vi "FA Values View2.vi"(11 "Model in":refnum<class "Model.lvclass">) -> ()   [LabVIEW 2016, in "M1M3SupportEUI_Views.lvlib"]
uses:
  M1M3SupportEUI_Views.lvlib
  Model/Model.lvclass
  SALLV_m1m3/DataTypes/ForceActuatorData.ctl
  SALLV_m1m3/DataTypes/logevent_ForceActuatorInfo.ctl
  SALLV_m1m3/DataTypes/logevent_ForceActuatorState.ctl
  SALLV_m1m3/DataTypes/logevent_ForceActuatorWarning.ctl
  SALLV_m1m3/DataTypes/logevent_ForceSetpointWarning.ctl
  SALLV_m1m3/DataTypes/logevent_ForceActuatorForceWarning.ctl
  SALLV_m1m3/DataTypes/logevent_AppliedAberrationForces.ctl
  SALLV_m1m3/DataTypes/logevent_AppliedAccelerationForces.ctl
  SALLV_m1m3/DataTypes/logevent_AppliedActiveOpticForces.ctl
  SALLV_m1m3/DataTypes/logevent_AppliedAzimuthForces.ctl
  SALLV_m1m3/DataTypes/logevent_AppliedBalanceForces.ctl
  SALLV_m1m3/DataTypes/logevent_AppliedCylinderForces.ctl
  SALLV_m1m3/DataTypes/logevent_AppliedElevationForces.ctl
  SALLV_m1m3/DataTypes/logevent_AppliedForces.ctl
  SALLV_m1m3/DataTypes/logevent_AppliedOffsetForces.ctl
  SALLV_m1m3/DataTypes/logevent_AppliedStaticForces.ctl
  SALLV_m1m3/DataTypes/logevent_AppliedThermalForces.ctl
  SALLV_m1m3/DataTypes/logevent_AppliedVelocityForces.ctl
  SALLV_m1m3/DataTypes/logevent_RejectedAberrationForces.ctl
  SALLV_m1m3/DataTypes/logevent_RejectedAccelerationForces.ctl
  SALLV_m1m3/DataTypes/logevent_RejectedActiveOpticForces.ctl
  SALLV_m1m3/DataTypes/logevent_RejectedAzimuthForces.ctl
  SALLV_m1m3/DataTypes/logevent_RejectedBalanceForces.ctl
  SALLV_m1m3/DataTypes/logevent_RejectedCylinderForces.ctl
  SALLV_m1m3/DataTypes/logevent_RejectedElevationForces.ctl
  SALLV_m1m3/DataTypes/logevent_RejectedForces.ctl
  SALLV_m1m3/DataTypes/logevent_RejectedOffsetForces.ctl
  SALLV_m1m3/DataTypes/logevent_RejectedStaticForces.ctl
  SALLV_m1m3/DataTypes/logevent_RejectedThermalForces.ctl
  SALLV_m1m3/DataTypes/logevent_RejectedVelocityForces.ctl
  M1M3 Support Events/M1M3 Support Events.lvclass/M1M3 Support Events.ctl
  M1M3 Support Events/M1M3 Support Events.lvclass
  SALLV_m1m3/SALLV_m1m3.lvlib
panel:
  out "Numeric":i32
  out "Timestamp":timestamp
  in  "logevent_RejectedVelocityForces":T1
  in  "logevent_RejectedThermalForces":T2
  in  "logevent_RejectedStaticForces":T3
  in  "logevent_RejectedOffsetForces":T4
  in  "logevent_RejectedForces":T5
  in  "logevent_RejectedElevationForces":T6
  in  "logevent_RejectedCylinderForces":T7
  in  "logevent_RejectedBalanceForces":T8
  in  "logevent_RejectedAzimuthForces":T9
  in  "logevent_RejectedActiveOpticForces":T10
  in  "logevent_RejectedAccelerationForces":T11
  in  "logevent_RejectedAberrationForces":T12
  in  "logevent_AppliedVelocityForces":T13
  in  "logevent_AppliedThermalForces":T14
  in  "logevent_AppliedStaticForces":T15
  in  "logevent_AppliedOffsetForces":T16
  in  "logevent_AppliedForces":T17
  in  "logevent_AppliedElevationForces":T18
  in  "logevent_AppliedCylinderForces":T19
  in  "logevent_AppliedBalanceForces":T20
  in  "logevent_AppliedAzimuthForces":T21
  in  "logevent_AppliedActiveOpticForces":T22
  in  "logevent_AppliedAccelerationForces":T23
  in  "logevent_AppliedAberrationForces":T24
  in  "logevent_ForceActuatorForceWarning":T25
  in  "logevent_ForceSetpointWarning":T26
  in  "logevent_ForceActuatorWarning":T27
  in  "logevent_ForceActuatorState":T28
  out "logevent_ForceActuatorInfo":T29
  out "ForceActuatorData":T30 {"Timestamp" format="%#_14f"}
  in  "Field":string(combo)
  out "Display":string[][](array[string])
  out "stop":bool
  in  "Topic":string(combo)
  # "Force Actuators"
  # "0"
  # "1"
  # "2"
  # "3"
  # "4"
  # "5"
  # "6"
  # "7"
  # "8"
  # "9"
  # "100"
  # "110"
  # "120"
  # "130"
  # "140"
  # "200"
  # "210"
  # "220"
  # "230"
  # "240"
  # "300"
  # "310"
  # "320"
  # "330"
  # "340"
  # "400"
  # "410"
  # "420"
  # "430"
  # "440"
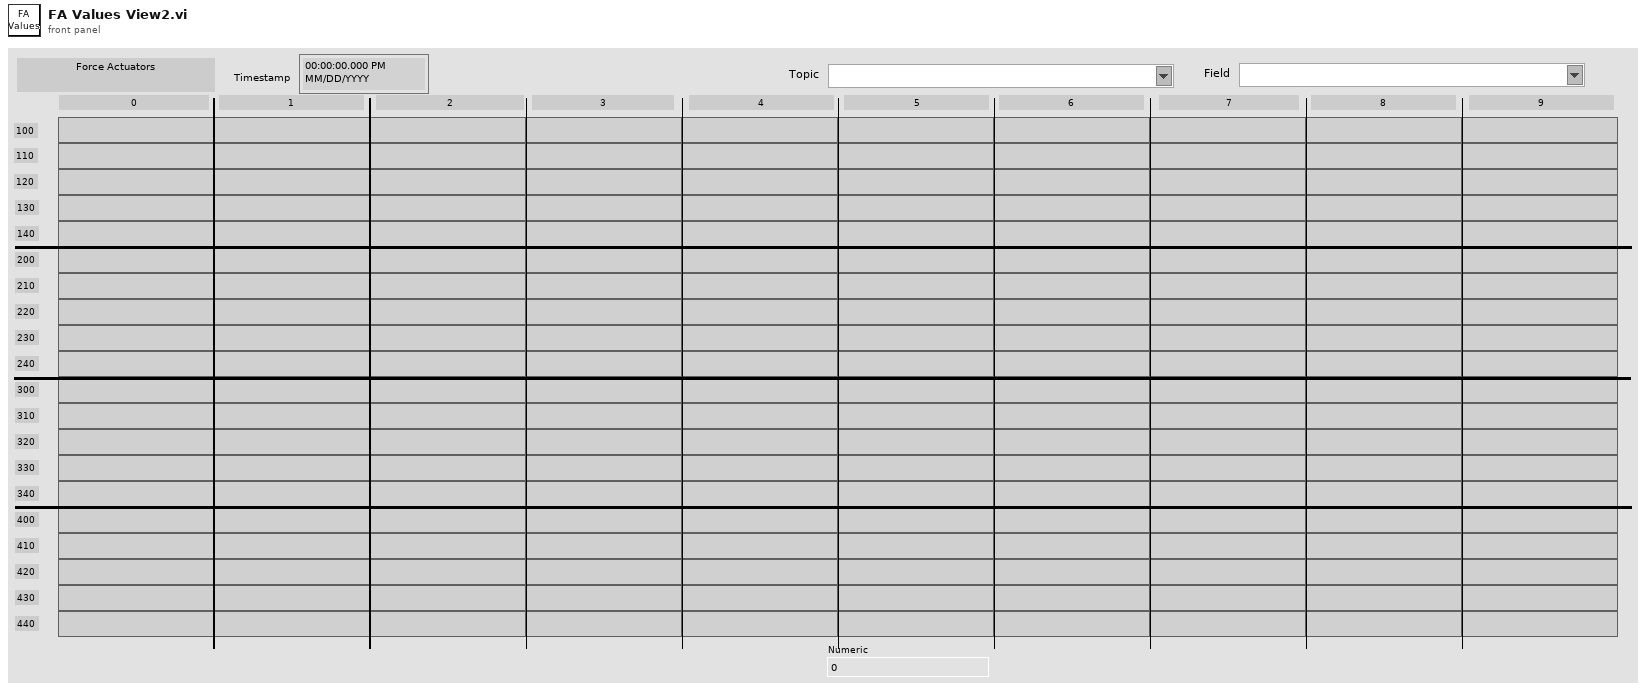
[diagram p1: front panel]
types:
  T1 = typedef "SALLV_m1m3.lvlib/logevent_RejectedVelocityForces.ctl" = cluster{"Timestamp":dbl, "XForces[12]":sgl[], "YForces[100]":sgl[], "ZForces[156]":sgl[], "Fx":sgl, "Fy":sgl, "Fz":sgl, "Mx":sgl, "My":sgl, "Mz":sgl, "ForceMagnitude":sgl, "priority":i32}
  T2 = typedef "SALLV_m1m3.lvlib/logevent_RejectedThermalForces.ctl" = cluster{"Timestamp":dbl, "XForces[12]":sgl[], "YForces[100]":sgl[], "ZForces[156]":sgl[], "Fx":sgl, "Fy":sgl, "Fz":sgl, "Mx":sgl, "My":sgl, "Mz":sgl, "ForceMagnitude":sgl, "priority":i32}
  T3 = typedef "SALLV_m1m3.lvlib/logevent_RejectedStaticForces.ctl" = cluster{"Timestamp":dbl, "XForces[12]":sgl[], "YForces[100]":sgl[], "ZForces[156]":sgl[], "Fx":sgl, "Fy":sgl, "Fz":sgl, "Mx":sgl, "My":sgl, "Mz":sgl, "ForceMagnitude":sgl, "priority":i32}
  T4 = typedef "SALLV_m1m3.lvlib/logevent_RejectedOffsetForces.ctl" = cluster{"Timestamp":dbl, "XForces[12]":sgl[], "YForces[100]":sgl[], "ZForces[156]":sgl[], "Fx":sgl, "Fy":sgl, "Fz":sgl, "Mx":sgl, "My":sgl, "Mz":sgl, "ForceMagnitude":sgl, "priority":i32}
  T5 = typedef "SALLV_m1m3.lvlib/logevent_RejectedForces.ctl" = cluster{"Timestamp":dbl, "XForces[12]":sgl[], "YForces[100]":sgl[], "ZForces[156]":sgl[], "Fx":sgl, "Fy":sgl, "Fz":sgl, "Mx":sgl, "My":sgl, "Mz":sgl, "ForceMagnitude":sgl, "priority":i32}
  T6 = typedef "SALLV_m1m3.lvlib/logevent_RejectedElevationForces.ctl" = cluster{"Timestamp":dbl, "XForces[12]":sgl[], "YForces[100]":sgl[], "ZForces[156]":sgl[], "Fx":sgl, "Fy":sgl, "Fz":sgl, "Mx":sgl, "My":sgl, "Mz":sgl, "ForceMagnitude":sgl, "priority":i32}
  T7 = typedef "SALLV_m1m3.lvlib/logevent_RejectedCylinderForces.ctl" = cluster{"Timestamp":dbl, "SecondaryCylinderForces[112]":i32[], "PrimaryCylinderForces[156]":i32[], "priority":i32}
  T8 = typedef "SALLV_m1m3.lvlib/logevent_RejectedBalanceForces.ctl" = cluster{"Timestamp":dbl, "XForces[12]":sgl[], "YForces[100]":sgl[], "ZForces[156]":sgl[], "Fx":sgl, "Fy":sgl, "Fz":sgl, "Mx":sgl, "My":sgl, "Mz":sgl, "ForceMagnitude":sgl, "priority":i32}
  T9 = typedef "SALLV_m1m3.lvlib/logevent_RejectedAzimuthForces.ctl" = cluster{"Timestamp":dbl, "XForces[12]":sgl[], "YForces[100]":sgl[], "ZForces[156]":sgl[], "Fx":sgl, "Fy":sgl, "Fz":sgl, "Mx":sgl, "My":sgl, "Mz":sgl, "ForceMagnitude":sgl, "priority":i32}
  T10 = typedef "SALLV_m1m3.lvlib/logevent_RejectedActiveOpticForces.ctl" = cluster{"Timestamp":dbl, "ZForces[156]":sgl[], "Fz":sgl, "Mx":sgl, "My":sgl, "priority":i32}
  T11 = typedef "SALLV_m1m3.lvlib/logevent_RejectedAccelerationForces.ctl" = cluster{"Timestamp":dbl, "XForces[12]":sgl[], "YForces[100]":sgl[], "ZForces[156]":sgl[], "Fx":sgl, "Fy":sgl, "Fz":sgl, "Mx":sgl, "My":sgl, "Mz":sgl, "ForceMagnitude":sgl, "priority":i32}
  T12 = typedef "SALLV_m1m3.lvlib/logevent_RejectedAberrationForces.ctl" = cluster{"Timestamp":dbl, "ZForces[156]":sgl[], "Fz":sgl, "Mx":sgl, "My":sgl, "priority":i32}
  T13 = typedef "SALLV_m1m3.lvlib/logevent_AppliedVelocityForces.ctl" = cluster{"Timestamp":dbl, "XForces[12]":sgl[], "YForces[100]":sgl[], "ZForces[156]":sgl[], "Fx":sgl, "Fy":sgl, "Fz":sgl, "Mx":sgl, "My":sgl, "Mz":sgl, "ForceMagnitude":sgl, "priority":i32}
  T14 = typedef "SALLV_m1m3.lvlib/logevent_AppliedThermalForces.ctl" = cluster{"Timestamp":dbl, "XForces[12]":sgl[], "YForces[100]":sgl[], "ZForces[156]":sgl[], "Fx":sgl, "Fy":sgl, "Fz":sgl, "Mx":sgl, "My":sgl, "Mz":sgl, "ForceMagnitude":sgl, "priority":i32}
  T15 = typedef "SALLV_m1m3.lvlib/logevent_AppliedStaticForces.ctl" = cluster{"Timestamp":dbl, "XForces[12]":sgl[], "YForces[100]":sgl[], "ZForces[156]":sgl[], "Fx":sgl, "Fy":sgl, "Fz":sgl, "Mx":sgl, "My":sgl, "Mz":sgl, "ForceMagnitude":sgl, "priority":i32}
  T16 = typedef "SALLV_m1m3.lvlib/logevent_AppliedOffsetForces.ctl" = cluster{"Timestamp":dbl, "XForces[12]":sgl[], "YForces[100]":sgl[], "ZForces[156]":sgl[], "Fx":sgl, "Fy":sgl, "Fz":sgl, "Mx":sgl, "My":sgl, "Mz":sgl, "ForceMagnitude":sgl, "priority":i32}
  T17 = typedef "SALLV_m1m3.lvlib/logevent_AppliedForces.ctl" = cluster{"Timestamp":dbl, "XForces[12]":sgl[], "YForces[100]":sgl[], "ZForces[156]":sgl[], "Fx":sgl, "Fy":sgl, "Fz":sgl, "Mx":sgl, "My":sgl, "Mz":sgl, "ForceMagnitude":sgl, "priority":i32}
  T18 = typedef "SALLV_m1m3.lvlib/logevent_AppliedElevationForces.ctl" = cluster{"Timestamp":dbl, "XForces[12]":sgl[], "YForces[100]":sgl[], "ZForces[156]":sgl[], "Fx":sgl, "Fy":sgl, "Fz":sgl, "Mx":sgl, "My":sgl, "Mz":sgl, "ForceMagnitude":sgl, "priority":i32}
  T19 = typedef "SALLV_m1m3.lvlib/logevent_AppliedCylinderForces.ctl" = cluster{"Timestamp":dbl, "SecondaryCylinderForces[112]":i32[], "PrimaryCylinderForces[156]":i32[], "priority":i32}
  T20 = typedef "SALLV_m1m3.lvlib/logevent_AppliedBalanceForces.ctl" = cluster{"Timestamp":dbl, "XForces[12]":sgl[], "YForces[100]":sgl[], "ZForces[156]":sgl[], "Fx":sgl, "Fy":sgl, "Fz":sgl, "Mx":sgl, "My":sgl, "Mz":sgl, "ForceMagnitude":sgl, "priority":i32}
  T21 = typedef "SALLV_m1m3.lvlib/logevent_AppliedAzimuthForces.ctl" = cluster{"Timestamp":dbl, "XForces[12]":sgl[], "YForces[100]":sgl[], "ZForces[156]":sgl[], "Fx":sgl, "Fy":sgl, "Fz":sgl, "Mx":sgl, "My":sgl, "Mz":sgl, "ForceMagnitude":sgl, "priority":i32}
  T22 = typedef "SALLV_m1m3.lvlib/logevent_AppliedActiveOpticForces.ctl" = cluster{"Timestamp":dbl, "ZForces[156]":sgl[], "Fz":sgl, "Mx":sgl, "My":sgl, "priority":i32}
  T23 = typedef "SALLV_m1m3.lvlib/logevent_AppliedAccelerationForces.ctl" = cluster{"Timestamp":dbl, "XForces[12]":sgl[], "YForces[100]":sgl[], "ZForces[156]":sgl[], "Fx":sgl, "Fy":sgl, "Fz":sgl, "Mx":sgl, "My":sgl, "Mz":sgl, "ForceMagnitude":sgl, "priority":i32}
  T24 = typedef "SALLV_m1m3.lvlib/logevent_AppliedAberrationForces.ctl" = cluster{"Timestamp":dbl, "ZForces[156]":sgl[], "Fz":sgl, "Mx":sgl, "My":sgl, "priority":i32}
  T25 = typedef "SALLV_m1m3.lvlib/logevent_ForceActuatorForceWarning.ctl" = cluster{"Timestamp":dbl, "AnyWarning":bool, "AnyPrimaryAxisMeasuredForceWarning":bool, "PrimaryAxisMeasuredForceWarning[156]":bool[], "AnySecondaryAxisMeasuredForceWarning":bool, "SecondaryAxisMeasuredForceWarning[156]":bool[], "AnyPrimaryAxisFollowingErrorWarning":bool, "PrimaryAxisFollowingErrorWarning[156]":bool[], "AnySecondaryAxisFollowingErrorWarning":bool, "SecondaryAxisFollowingErrorWarning[156]":bool[], "priority":i32}
  T26 = typedef "SALLV_m1m3.lvlib/logevent_ForceSetpointWarning.ctl" = cluster{"Timestamp":dbl, "AnyWarning":bool, "AnySafetyLimitWarning":bool, "SafetyLimitWarning[156]":bool[], "XMomentWarning":bool, "YMomentWarning":bool, "ZMomentWarning":bool, "AnyNearNeighborWarning":bool, "NearNeighborWarning[156]":bool[], "MagnitudeWarning":bool, "AnyFarNeighborWarning":bool, "FarNeighborWarning[156]":bool[], "AnyElevationForceWarning":bool, "ElevationForceWarning[156]":bool[], "AnyAzimuthForceWarning":bool, "AzimuthForceWarning[156]":bool[], "AnyThermalForceWarning":bool, "ThermalForceWarning[156]":bool[], "AnyBalanceForceWarning":bool, "BalanceForceWarning[156]":bool[], "AnyAccelerationForceWarning":bool, "AccelerationForceWarning[156]":bool[], "ActiveOpticNetForceWarning":bool, "AnyActiveOpticForceWarning":bool, "ActiveOpticForceWarning[156]":bool[], "AnyStaticForceWarning":bool, "StaticForceWarning[156]":bool[], "AberrationNetForceWarning":bool, "AnyAberrationForceWarning":bool, "AberrationForceWarning[156]":bool[], "AnyOffsetForceWarning":bool, "OffsetForceWarning[156]":bool[], "AnyVelocityForceWarning":bool, "VelocityForceWarning[156]":bool[], "AnyForceWarning":bool, "ForceWarning[156]":bool[], "priority":i32}
  T27 = typedef "SALLV_m1m3.lvlib/logevent_ForceActuatorWarning.ctl" = cluster{"Timestamp":dbl, "AnyWarning":bool, "AnyMajorFault":bool, "MajorFault[156]":bool[], "AnyMinorFault":bool, "MinorFault[156]":bool[], "AnyFaultOverride":bool, "FaultOverride[156]":bool[], "AnyMainCalibrationError":bool, "MainCalibrationError[156]":bool[], "AnyBackupCalibrationError":bool, "BackupCalibrationError[156]":bool[], "AnyMezzanineError":bool, "MezzanineError[156]":bool[], "AnyMezzanineBootloaderActive":bool, "MezzanineBootloaderActive[156]":bool[], "AnyUniqueIdCRCError":bool, "UniqueIdCRCError[156]":bool[], "AnyApplicationTypeMismatch":bool, "ApplicationTypeMismatch[156]":bool[], "AnyApplicationMissing":bool, "ApplicationMissing[156]":bool[], "AnyApplicationCRCMismatch":bool, "ApplicationCRCMismatch[156]":bool[], "AnyOneWireMissing":bool, "OneWireMissing[156]":bool[], "AnyOneWire1Mismatch":bool, "OneWire1Mismatch[156]":bool[], "AnyOneWire2Mismatch":bool, "OneWire2Mismatch[156]":bool[], "AnyWatchdogReset":bool, "WatchdogReset[156]":bool[], "AnyBrownOut":bool, "BrownOut[156]":bool[], "AnyEventTrapReset":bool, "EventTrapReset[156]":bool[], "AnySSRPowerFault":bool, "SSRPowerFault[156]":bool[], "AnyAuxPowerFault":bool, "AuxPowerFault[156]":bool[], "AnyMezzaninePowerFault":bool, "MezzaninePowerFault[156]":bool[], "AnyMezzanineCurrentAmp1Fault":bool, "MezzanineCurrentAmp1Fault[156]":bool[], "AnyMezzanineCurrentAmp2Fault":bool, "MezzanineCurrentAmp2Fault[156]":bool[], "AnyMezzanineUniqueIdCRCError":bool, "MezzanineUniqueIdCRCError[156]":bool[], "AnyMezzanineMainCalibrationError":bool, "MezzanineMainCalibrationError[156]":bool[], "AnyMezzanineBackupCalibrationError":bool, "MezzanineBackupCalibrationError[156]":bool[], "AnyMezzanineEventTrapReset":bool, "MezzanineEventTrapReset[156]":bool[], "AnyMezzanineApplicationMissing":bool, "MezzanineApplicationMissing[156]":bool[], "AnyMezzanineApplicationCRCMismatch":bool, "MezzanineApplicationCRCMismatch[156]":bool[], "AnyILCFault":bool, "ILCFault[156]":bool[], "AnyBroadcastCounterWarning":bool, "BroadcastCounterWarning[156]":bool[], "priority":i32}
  T28 = typedef "SALLV_m1m3.lvlib/logevent_ForceActuatorState.ctl" = cluster{"Timestamp":dbl, "ILCState[156]":i16[], "SlewFlag":bool, "StaticForcesApplied":bool, "ElevationForcesApplied":bool, "AzimuthForcesApplied":bool, "ThermalForcesApplied":bool, "OffsetForcesApplied":bool, "AccelerationForcesApplied":bool, "VelocityForcesApplied":bool, "ActiveOpticForcesApplied":bool, "AberrationForcesApplied":bool, "BalanceForcesApplied":bool, "SupportPercentage":sgl, "priority":i32}
  T29 = typedef "SALLV_m1m3.lvlib/logevent_ForceActuatorInfo.ctl" = cluster{"Timestamp":dbl, "ReferenceId[156]":i16[], "XDataReferenceId[12]":i16[], "YDataReferenceId[100]":i16[], "ZDataReferenceId[156]":i16[], "ActuatorType[156]":i16[], "ActuatorOrientation[156]":i16[], "ModbusSubnet[156]":i16[], "ModbusAddress[156]":i16[], "XPosition[156]":sgl[], "YPosition[156]":sgl[], "ZPosition[156]":sgl[], "ILCUniqueId[156]":i64[], "ILCApplicationType[156]":i16[], "NetworkNodeType[156]":i16[], "ILCSelectedOptions[156]":i16[], "NetworkNodeOptions[156]":i16[], "MajorRevision[156]":i16[], "MinorRevision[156]":i16[], "ADCScanRate[156]":i16[], "MainPrimaryCylinderCoefficient[156]":sgl[], "MainSecondaryCylinderCoefficient[156]":sgl[], "MainPrimaryCylinderLoadCellOffset[156]":sgl[], "MainSecondaryCylinderLoadCellOffset[156]":sgl[], "MainPrimaryCylinderLoadCellSensitivity[156]":sgl[], "MainSecondaryCylinderLoadCellSensitivity[156]":sgl[], "BackupPrimaryCylinderCoefficient[156]":sgl[], "BackupSecondaryCylinderCoefficient[156]":sgl[], "BackupPrimaryCylinderLoadCellOffset[156]":sgl[], "BackupSecondaryCylinderLoadCellOffset[156]":sgl[], "BackupPrimaryCylinderLoadCellSensitivity[156]":sgl[], "BackupSecondaryCylinderLoadCellSensitivity[156]":sgl[], "MezzaninePrimaryCylinderGain[156]":sgl[], "MezzanineSecondaryCylinderGain[156]":sgl[], "MezzanineUniqueId[156]":i64[], "MezzanineFirmwareType[156]":i16[], "MezzanineMajorRevision[156]":i16[], "MezzanineMinorRevision[156]":i16[], "priority":i32}
  T30 = typedef "SALLV_m1m3.lvlib/ForceActuatorData.ctl" = cluster{"Timestamp":dbl, "PrimaryCylinderForce[156]":sgl[], "SecondaryCylinderForce[112]":sgl[], "XForce[12]":sgl[], "YForce[100]":sgl[], "ZForce[156]":sgl[], "Fx":sgl, "Fy":sgl, "Fz":sgl, "Mx":sgl, "My":sgl, "Mz":sgl, "ForceMagnitude":sgl}
  T31 = typedef "M1M3SupportEUI_TypeDefs.lvlib/M1M3 Support Events.ctl" = cluster{"Inclinometer  Data":refnum<user-event>, "IMS Data":refnum<user-event>, "SAL Connected":refnum<user-event>, "Accelerometer Data":refnum<user-event>, "OuterLoop Data":refnum<user-event>, "ErrorCode Event":refnum<user-event>, "InterlockStatus Event":refnum<user-event>, "InterlockWarning Event":refnum<user-event>, "Gyro Data":refnum<user-event>, "HP Actuator Info Event":refnum<user-event>, " FA Info Event":refnum<user-event>, "HP Monitor Info Event":refnum<user-event>, "FA Data":refnum<user-event>, "HP Actuator data":refnum<user-event>, "HP Monitor data":refnum<user-event>, "Air Supply Status Event":refnum<user-event>, "Air Supply Warning Event":refnum<user-event>, "Power Data":refnum<user-event>, "PID Data":refnum<user-event>, "PID Info Event":refnum<user-event>, "Power Status Event":refnum<user-event>, "Power Supply Status Event":refnum<user-event>, "Power Warning Event":refnum<user-event>, "Summary State Event":refnum<user-event>, "Detailed State Event":refnum<user-event>, "FA Force Warning Event":refnum<user-event>, "FA Warning Event":refnum<user-event>, "FA State Event":refnum<user-event>, "Applied AberrationForces Event":refnum<user-event>, "Applied Acceleration Forcces Event":refnum<user-event>, "Applied Azimuth Forces Event":refnum<user-event>, "Applied Active Optic Forces Event":refnum<user-event>, "Applied Balance Forces Event":refnum<user-event>, "Applied Cylinder Forces Event":refnum<user-event>, "Applied Elevation Forces Event":refnum<user-event>, "Applied Forces Event":refnum<user-event>, "Applied Offset Forces Event":refnum<user-event>, "Applied Static Forces Event":refnum<user-event>, "Applied Thermal Forces Event":refnum<user-event>, "Applied Velocity Forces Event":refnum<user-event>, "Rejected Aberration Force Event":refnum<user-event>, "Rejected Acceleration Forces Event":refnum<user-event>, "Rejected Active Optic Forces Event":refnum<user-event>, "Rejected Azimuth Forces Event":refnum<user-event>, "Rejected Balance Forces Event":refnum<user-event>, "Rejected Cylinder Forces Event":refnum<user-event>, "Rejected Elevation Forces Event":refnum<user-event>, "Rejected Forces Event":refnum<user-event>, "Rejected Offset Forces Event":refnum<user-event>, "Rejected Static Forces Event":refnum<user-event>, "Rejected Thermal Forces Event":refnum<user-event>, "Rejected Velocity Forces Event":refnum<user-event>, "Command Rejection Event":refnum<user-event>, "Setting Verions Event":refnum<user-event>, "Settings Applied Event":refnum<user-event>, "HP Actuator State Event":refnum<user-event>, "HP Actuator Warning Event":refnum<user-event>, "HP Monitor State Event":refnum<user-event>, "HP Monitor Warning Event":refnum<user-event>, "Accelerometer Warning Event":refnum<user-event>, "Applied Settings Match Start Event":refnum<user-event>, "Cell Light Status Event ":refnum<user-event>, "Cell Light Warning Event":refnum<user-event>, "Displacement Sensor Warning Event":refnum<user-event>, "Force Setpoint Warning Event":refnum<user-event>, "Gyro Warning Event ":refnum<user-event>, "ILC Warning Event ":refnum<user-event>, "Inclinometer Sensor Warning Event ":refnum<user-event>}
  T32 = enum16{"", "DetailedState_DetailedStates_DisabledState", "DetailedState_DetailedStates_EnabledState", "DetailedState_DetailedStates_FaultState", "DetailedState_DetailedStates_OfflineState", "DetailedState_DetailedStates_StandbyState", "DetailedState_DetailedStates_ParkedState", "DetailedState_DetailedStates_RaisingState", "DetailedState_DetailedStates_ActiveState", "DetailedState_DetailedStates_LoweringState", "DetailedState_DetailedStates_EngineeringState", "DetailedState_DetailedStates_ParkedEngineeringState", "DetailedState_DetailedStates_RaisingEngineeringState", "DetailedState_DetailedStates_ActiveEngineeringState", "DetailedState_DetailedStates_LoweringEngineeringState", "DetailedState_DetailedStates_LoweringFaultState", "DetailedState_DetailedStates_ProfileHardpointCorrectionState"}
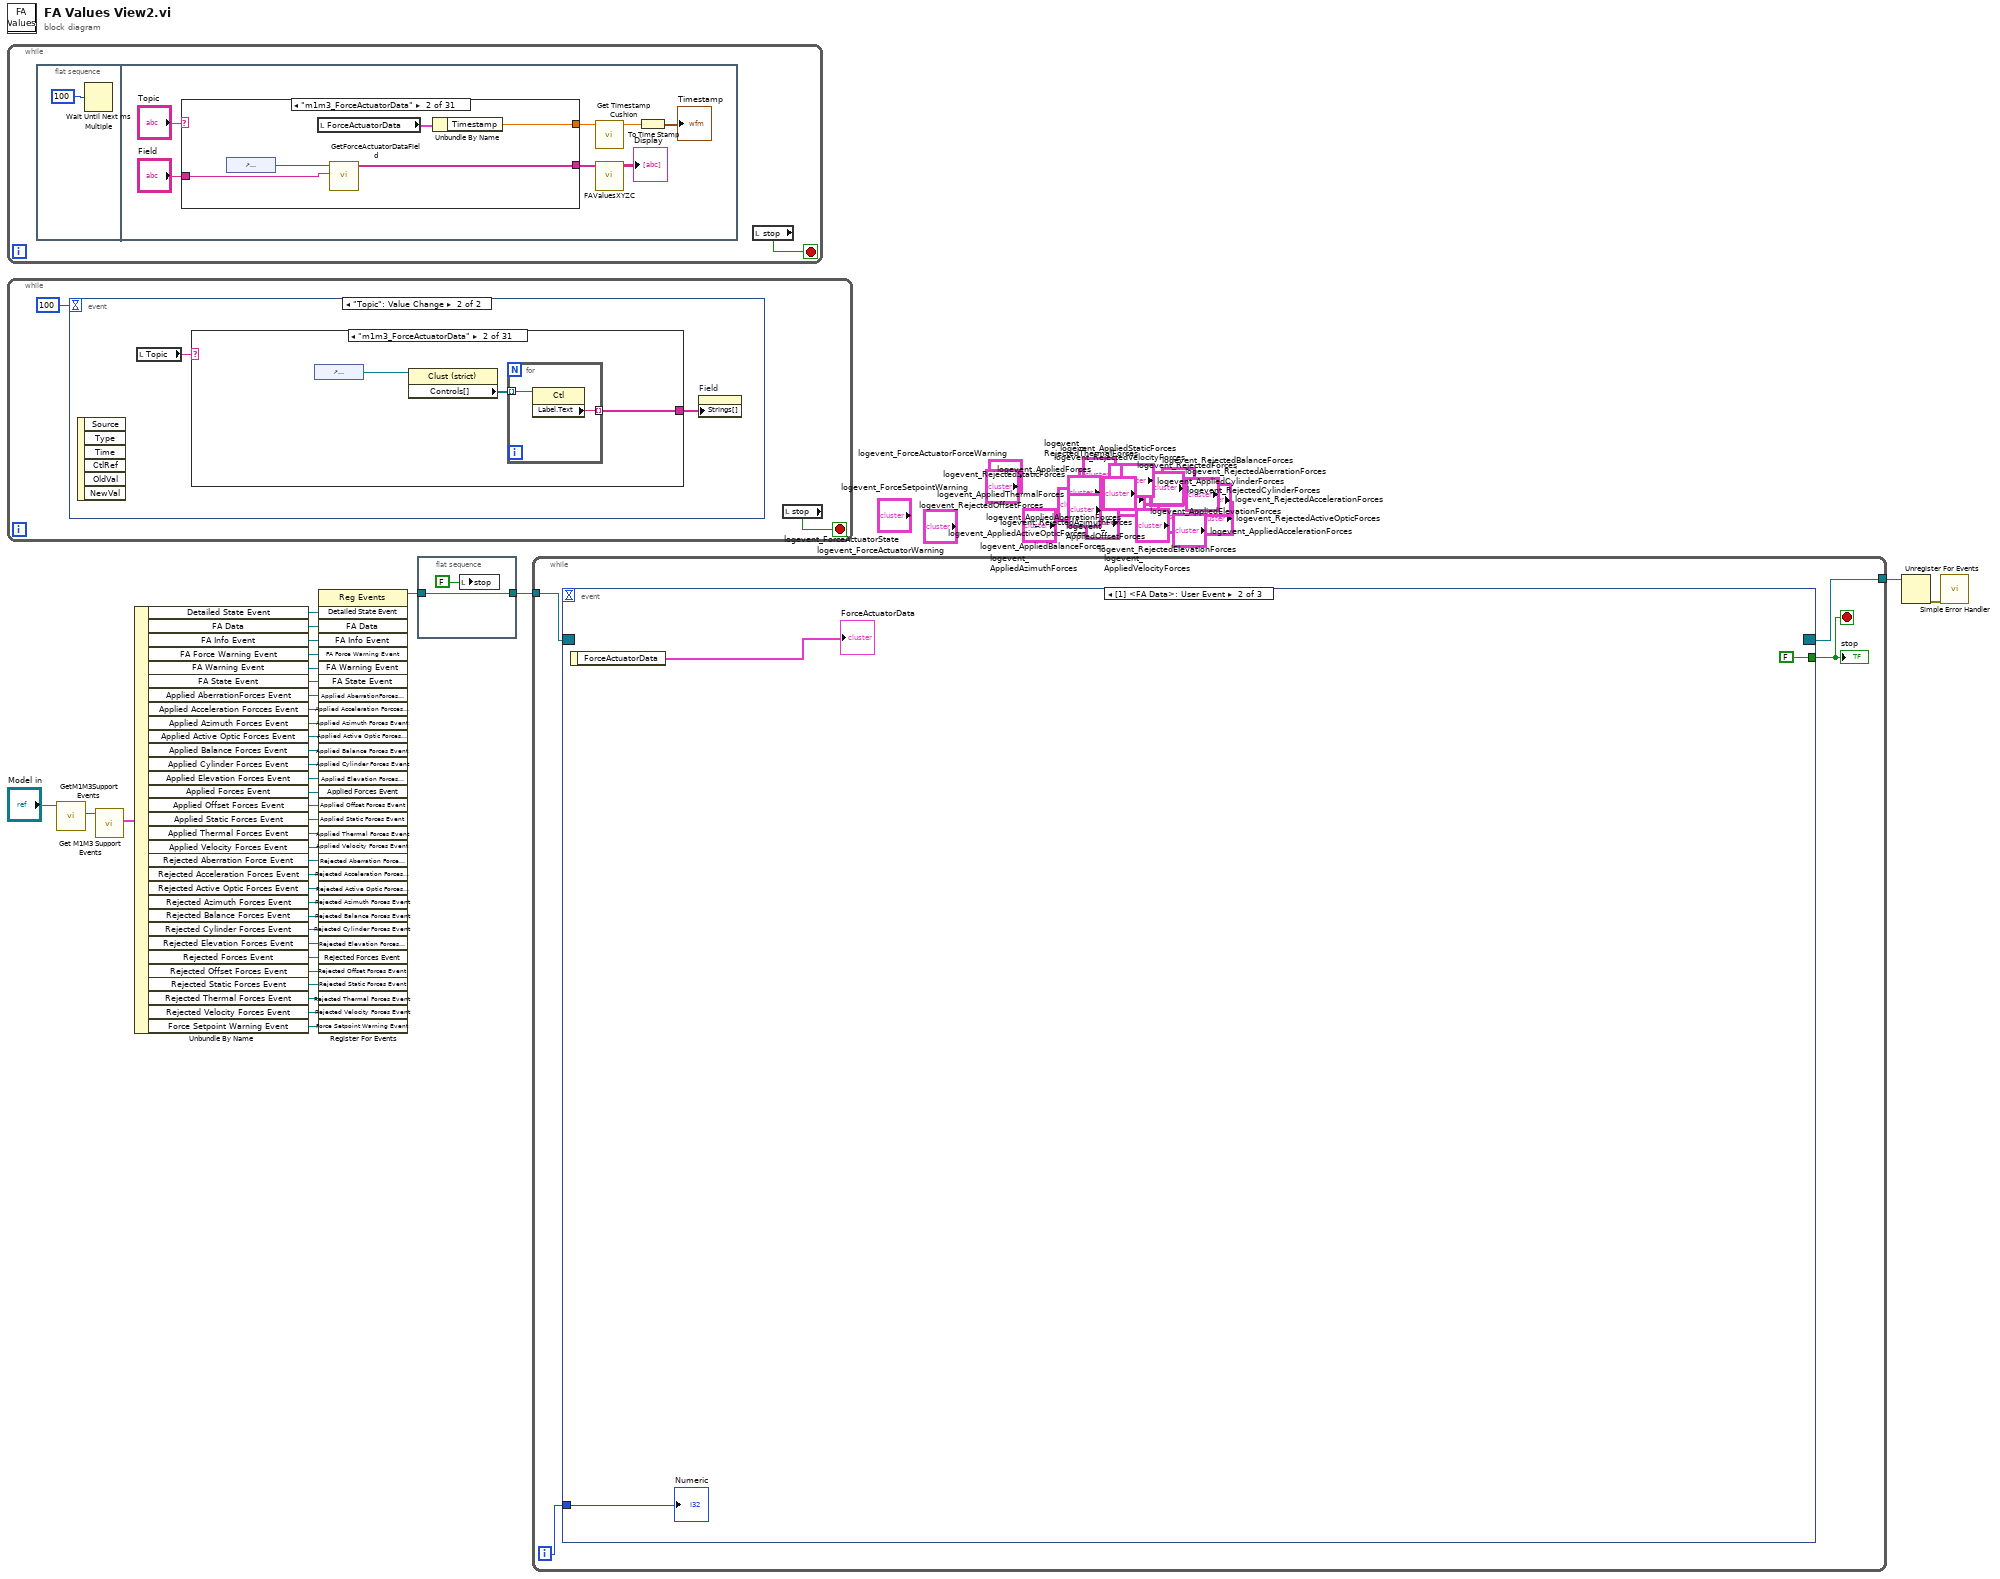
[diagram p0: block diagram]
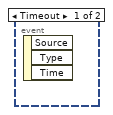
[diagram p2: hidden frame]
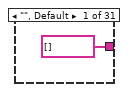
[diagram p3: hidden frame]
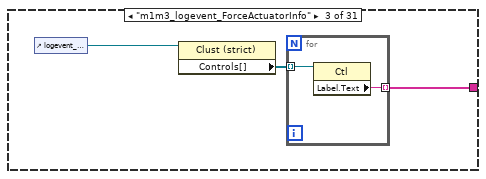
[diagram p4: hidden frame]
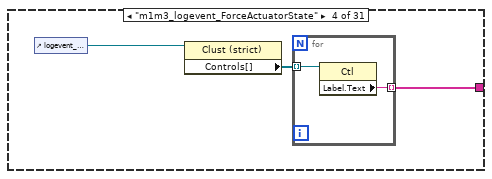
[diagram p5: hidden frame]
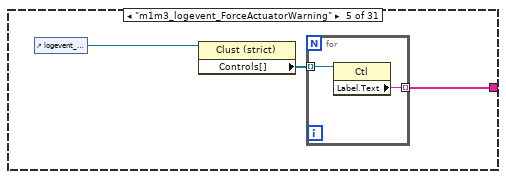
[diagram p6: hidden frame]
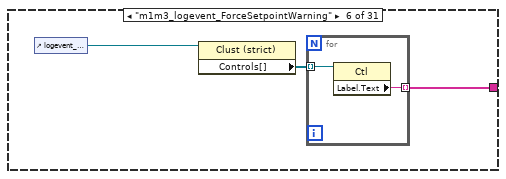
[diagram p7: hidden frame]
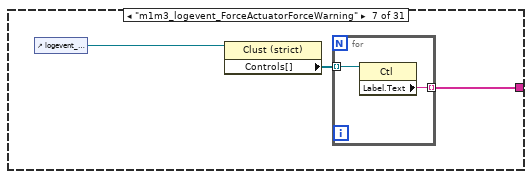
[diagram p8: hidden frame]
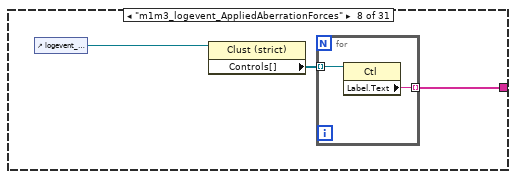
[diagram p9: hidden frame]
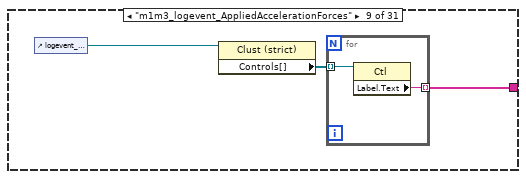
[diagram p10: hidden frame]
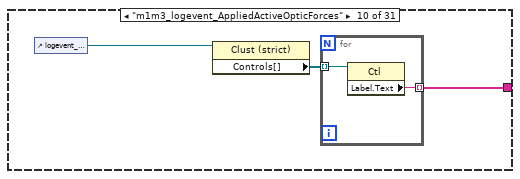
[diagram p11: hidden frame]
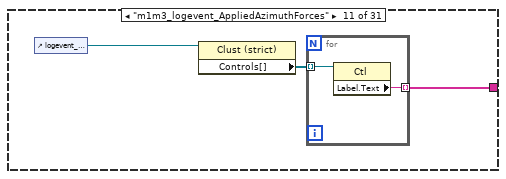
[diagram p12: hidden frame]
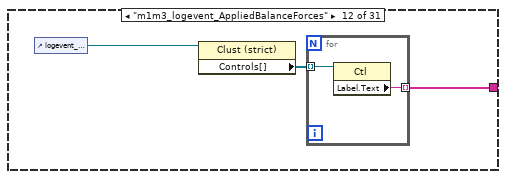
[diagram p13: hidden frame]
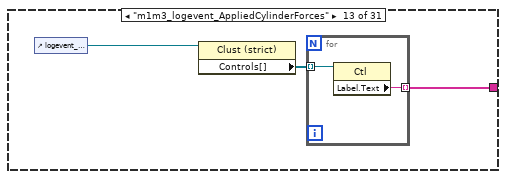
[diagram p14: hidden frame]
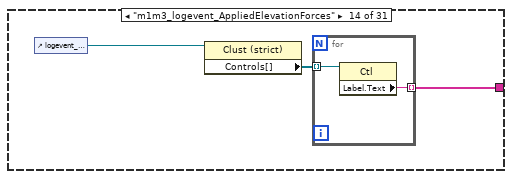
[diagram p15: hidden frame]
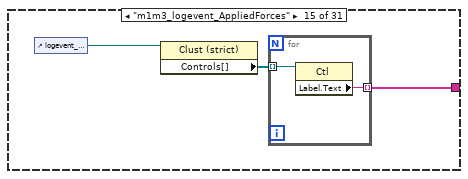
[diagram p16: hidden frame]
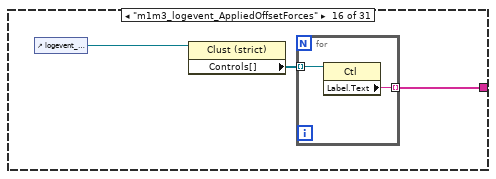
[diagram p17: hidden frame]
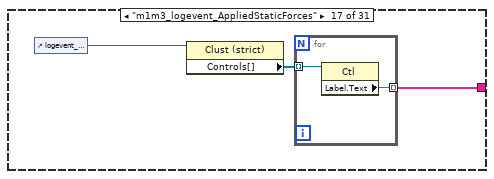
[diagram p18: hidden frame]
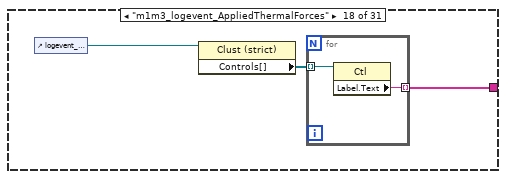
[diagram p19: hidden frame]
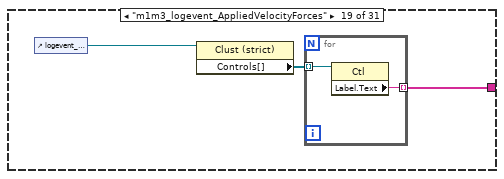
[diagram p20: hidden frame]
diagram:
  n1 = while {
    stop <- w39 stop-if-true
    n2 = flat-sequence {
      frame #0 {
        n3 = Wait Until Next ms Multiple(millisecond multiple=u32 100) -> ()  [unwired: 1 out]
      }
      frame #1 {
        n4 = case shown="\"m1m3_ForceActuatorData\"" "Topic" {
          tunnel: "Field" -> [_ w53 w58 w63 w68 w73 w77 w83 w88 w93 w98 w103 w108 w113 w118 w123 w128 w133 w138 w143 w148 w152 w158 w163 w168 w173 w178 w183 w188 w192 w198]
          tunnel: [string[] [] ("Array") w52 w57 w62 w67 w72 w78 w82 w87 w92 w97 w102 w107 w112 w117 w122 w127 w132 w137 w142 w147 w153 w157 w162 w167 w172 w177 w182 w187 w193 w197] -> w45
          tunnel: [0.0 w50 w55 w60 w65 w70 w75 w80 w85 w90 w95 w100 w105 w110 w115 w120 w125 w130 w135 w140 w145 w150 w155 w160 w165 w170 w175 w180 w185 w190 w195] -> w43
          frame "", Default {
          }
          frame "m1m3_ForceActuatorData" {
            n5 = control-ref of="ForceActuatorData"() -> (w54:refnum<vi>)
            n6 = local read "ForceActuatorData"() -> (w51:T30)
            n7 = call "GetForceActuatorDataField.vi"("Telemetry Data"=w53, "Cluster in"=w54) -> ("Array"=w52:string[])  [unwired: 9 in]
            n8 = Unbundle By Name(w51) -> ("Timestamp"=w50:dbl)
          }
          frame "m1m3_logevent_ForceActuatorInfo" {
            n9 = control-ref of="logevent_ForceActuatorInfo"() -> (w59:refnum<vi>)
            n10 = local read "logevent_ForceActuatorInfo"() -> (w56:T29)
            n11 = call "GetEventForceActuatorInfoField.vi"("Event Data"=w58, "Cluster in"=w59) -> ("Array"=w57:string[])  [unwired: 9 in]
            n12 = Unbundle By Name(w56) -> ("Timestamp"=w55:dbl)
          }
          frame "m1m3_logevent_ForceActuatorState" {
            n13 = control-ref of="logevent_ForceActuatorState"() -> (w64:refnum<vi>)
            n14 = local read "logevent_ForceActuatorState"() -> (w61:T28)
            n15 = call "GetEventForceActuatorStateField.vi"("Event Data"=w63, "Cluster in"=w64) -> ("Array"=w62:string[])  [unwired: 9 in]
            n16 = Unbundle By Name(w61) -> ("Timestamp"=w60:dbl)
          }
          frame "m1m3_logevent_ForceActuatorWarning" {
            n17 = control-ref of="logevent_ForceActuatorWarning"() -> (w69:refnum<vi>)
            n18 = local read "logevent_ForceActuatorWarning"() -> (w66:T27)
            n19 = call "GetEventForceActuatorWarningField.vi"("Event Data"=w68, "Cluster in"=w69) -> ("Array"=w67:string[])  [unwired: 9 in]
            n20 = Unbundle By Name(w66) -> ("Timestamp"=w65:dbl)
          }
          frame "m1m3_logevent_ForceSetpointWarning" {
            n21 = control-ref of="logevent_ForceSetpointWarning"() -> (w74:refnum<vi>)
            n22 = local read "logevent_ForceSetpointWarning"() -> (w71:T26)
            n23 = call "GetEventForceSetpointWarningField.vi"("Event Data"=w73, "Cluster in"=w74) -> ("Array"=w72:string[])  [unwired: 9 in]
            n24 = Unbundle By Name(w71) -> ("Timestamp"=w70:dbl)
          }
          frame "m1m3_logevent_ForceActuatorForceWarning" {
            n25 = local read "logevent_ForceActuatorForceWarning"() -> (w76:T25)
            n26 = control-ref of="logevent_ForceActuatorForceWarning"() -> (w79:refnum<vi>)
            n27 = Unbundle By Name(w76) -> ("Timestamp"=w75:dbl)
            n28 = call "GetEventForceActuatorForceWarningField.vi"("Event Data"=w77, "Cluster in"=w79) -> ("Array"=w78:string[])  [unwired: 9 in]
          }
          frame "m1m3_logevent_AppliedAberrationForces" {
            n29 = control-ref of="logevent_AppliedAberrationForces"() -> (w84:refnum<vi>)
            n30 = local read "logevent_AppliedAberrationForces"() -> (w81:T24)
            n31 = call "GetEventAppliedAberrationForcesField.vi"("Event Data"=w83, "Cluster in"=w84) -> ("Array"=w82:string[])  [unwired: 9 in]
            n32 = Unbundle By Name(w81) -> ("Timestamp"=w80:dbl)
          }
          frame "m1m3_logevent_AppliedAccelerationForces" {
            n33 = local read "logevent_AppliedAccelerationForces"() -> (w86:T23)
            n34 = control-ref of="logevent_AppliedAccelerationForces"() -> (w89:refnum<vi>)
            n35 = Unbundle By Name(w86) -> ("Timestamp"=w85:dbl)
            n36 = call "GetEventAppliedAccelerationForcesField.vi"("Event Data"=w88, "Cluster in"=w89) -> ("Array"=w87:string[])  [unwired: 9 in]
          }
          frame "m1m3_logevent_AppliedActiveOpticForces" {
            n37 = control-ref of="logevent_AppliedActiveOpticForces"() -> (w94:refnum<vi>)
            n38 = local read "logevent_AppliedActiveOpticForces"() -> (w91:T22)
            n39 = call "GetEventAppliedActiveOpticForcesField.vi"("Event Data"=w93, "Cluster in"=w94) -> ("Array"=w92:string[])  [unwired: 9 in]
            n40 = Unbundle By Name(w91) -> ("Timestamp"=w90:dbl)
          }
          frame "m1m3_logevent_AppliedAzimuthForces" {
            n41 = control-ref of="logevent_AppliedAzimuthForces"() -> (w99:refnum<vi>)
            n42 = local read "logevent_AppliedAzimuthForces"() -> (w96:T21)
            n43 = call "GetEventAppliedAzimuthForcesField.vi"("Event Data"=w98, "Cluster in"=w99) -> ("Array"=w97:string[])  [unwired: 9 in]
            n44 = Unbundle By Name(w96) -> ("Timestamp"=w95:dbl)
          }
          frame "m1m3_logevent_AppliedBalanceForces" {
            n45 = control-ref of="logevent_AppliedBalanceForces"() -> (w104:refnum<vi>)
            n46 = local read "logevent_AppliedBalanceForces"() -> (w101:T20)
            n47 = call "GetEventAppliedBalanceForcesField.vi"("Event Data"=w103, "Cluster in"=w104) -> ("Array"=w102:string[])  [unwired: 9 in]
            n48 = Unbundle By Name(w101) -> ("Timestamp"=w100:dbl)
          }
          frame "m1m3_logevent_AppliedCylinderForces" {
            n49 = control-ref of="logevent_AppliedCylinderForces"() -> (w109:refnum<vi>)
            n50 = local read "logevent_AppliedCylinderForces"() -> (w106:T19)
            n51 = call "GetEventAppliedCylinderForcesField.vi"("Event Data"=w108, "Cluster in"=w109) -> ("Array"=w107:string[])  [unwired: 9 in]
            n52 = Unbundle By Name(w106) -> ("Timestamp"=w105:dbl)
          }
          frame "m1m3_logevent_AppliedElevationForces" {
            n53 = control-ref of="logevent_AppliedElevationForces"() -> (w114:refnum<vi>)
            n54 = local read "logevent_AppliedElevationForces"() -> (w111:T18)
            n55 = call "GetEventAppliedElevationForcesField.vi"("Event Data"=w113, "Cluster in"=w114) -> ("Array"=w112:string[])  [unwired: 9 in]
            n56 = Unbundle By Name(w111) -> ("Timestamp"=w110:dbl)
          }
          frame "m1m3_logevent_AppliedForces" {
            n57 = control-ref of="logevent_AppliedForces"() -> (w119:refnum<vi>)
            n58 = local read "logevent_AppliedForces"() -> (w116:T17)
            n59 = call "GetEventAppliedForcesField.vi"("Event Data"=w118, "Cluster in"=w119) -> ("Array"=w117:string[])  [unwired: 9 in]
            n60 = Unbundle By Name(w116) -> ("Timestamp"=w115:dbl)
          }
          frame "m1m3_logevent_AppliedOffsetForces" {
            n61 = control-ref of="logevent_AppliedOffsetForces"() -> (w124:refnum<vi>)
            n62 = local read "logevent_AppliedOffsetForces"() -> (w121:T16)
            n63 = call "GetEventAppliedOffsetForcesField.vi"("Event Data"=w123, "Cluster in"=w124) -> ("Array"=w122:string[])  [unwired: 9 in]
            n64 = Unbundle By Name(w121) -> ("Timestamp"=w120:dbl)
          }
          frame "m1m3_logevent_AppliedStaticForces" {
            n65 = control-ref of="logevent_AppliedStaticForces"() -> (w129:refnum<vi>)
            n66 = local read "logevent_AppliedStaticForces"() -> (w126:T15)
            n67 = call "GetEventAppliedStaticForcesField.vi"("Event Data"=w128, "Cluster in"=w129) -> ("Array"=w127:string[])  [unwired: 9 in]
            n68 = Unbundle By Name(w126) -> ("Timestamp"=w125:dbl)
          }
          frame "m1m3_logevent_AppliedThermalForces" {
            n69 = control-ref of="logevent_AppliedThermalForces"() -> (w134:refnum<vi>)
            n70 = local read "logevent_AppliedThermalForces"() -> (w131:T14)
            n71 = call "GetEventAppliedThermalForcesField.vi"("Event Data"=w133, "Cluster in"=w134) -> ("Array"=w132:string[])  [unwired: 9 in]
            n72 = Unbundle By Name(w131) -> ("Timestamp"=w130:dbl)
          }
          frame "m1m3_logevent_AppliedVelocityForces" {
            n73 = control-ref of="logevent_AppliedVelocityForces"() -> (w139:refnum<vi>)
            n74 = local read "logevent_AppliedVelocityForces"() -> (w136:T13)
            n75 = call "GetEventAppliedVelocityForcesField.vi"("Event Data"=w138, "Cluster in"=w139) -> ("Array"=w137:string[])  [unwired: 9 in]
            n76 = Unbundle By Name(w136) -> ("Timestamp"=w135:dbl)
          }
          frame "m1m3_logevent_RejectedAberrationForces" {
            n77 = local read "logevent_RejectedAberrationForces"() -> (w141:T12)
            n78 = control-ref of="logevent_RejectedAberrationForces"() -> (w144:refnum<vi>)
            n79 = Unbundle By Name(w141) -> ("Timestamp"=w140:dbl)
            n80 = call "GetEventRejectedAberrationForcesField.vi"("Event Data"=w143, "Cluster in"=w144) -> ("Array"=w142:string[])  [unwired: 9 in]
          }
          frame "m1m3_logevent_RejectedAccelerationForces" {
            n81 = local read "logevent_RejectedAccelerationForces"() -> (w146:T11)
            n82 = control-ref of="logevent_RejectedAccelerationForces"() -> (w149:refnum<vi>)
            n83 = Unbundle By Name(w146) -> ("Timestamp"=w145:dbl)
            n84 = call "GetEventRejectedAccelerationForcesField.vi"("Event Data"=w148, "Cluster in"=w149) -> ("Array"=w147:string[])  [unwired: 9 in]
          }
          frame "m1m3_logevent_RejectedActiveOpticForces" {
            n85 = local read "logevent_RejectedActiveOpticForces"() -> (w151:T10)
            n86 = control-ref of="logevent_RejectedActiveOpticForces"() -> (w154:refnum<vi>)
            n87 = Unbundle By Name(w151) -> ("Timestamp"=w150:dbl)
            n88 = call "GetEventRejectedActiveOpticForcesField.vi"("Event Data"=w152, "Cluster in"=w154) -> ("Array"=w153:string[])  [unwired: 9 in]
          }
          frame "m1m3_logevent_RejectedAzimuthForces" {
            n89 = control-ref of="logevent_RejectedAzimuthForces"() -> (w159:refnum<vi>)
            n90 = local read "logevent_RejectedAzimuthForces"() -> (w156:T9)
            n91 = call "GetEventRejectedAzimuthForcesField.vi"("Event Data"=w158, "Cluster in"=w159) -> ("Array"=w157:string[])  [unwired: 9 in]
            n92 = Unbundle By Name(w156) -> ("Timestamp"=w155:dbl)
          }
          frame "m1m3_logevent_RejectedBalanceForces" {
            n93 = control-ref of="logevent_RejectedBalanceForces"() -> (w164:refnum<vi>)
            n94 = local read "logevent_RejectedBalanceForces"() -> (w161:T8)
            n95 = call "GetEventRejectedBalanceForcesField.vi"("Event Data"=w163, "Cluster in"=w164) -> ("Array"=w162:string[])  [unwired: 9 in]
            n96 = Unbundle By Name(w161) -> ("Timestamp"=w160:dbl)
          }
          frame "m1m3_logevent_RejectedCylinderForces" {
            n97 = control-ref of="logevent_RejectedCylinderForces"() -> (w169:refnum<vi>)
            n98 = local read "logevent_RejectedCylinderForces"() -> (w166:T7)
            n99 = call "GetEventRejectedCylinderForcesField.vi"("Event Data"=w168, "Cluster in"=w169) -> ("Array"=w167:string[])  [unwired: 9 in]
            n100 = Unbundle By Name(w166) -> ("Timestamp"=w165:dbl)
          }
          frame "m1m3_logevent_RejectedElevationForces" {
            n101 = control-ref of="logevent_RejectedElevationForces"() -> (w174:refnum<vi>)
            n102 = local read "logevent_RejectedElevationForces"() -> (w171:T6)
            n103 = call "GetEventRejectedElevationForcesField.vi"("Event Data"=w173, "Cluster in"=w174) -> ("Array"=w172:string[])  [unwired: 9 in]
            n104 = Unbundle By Name(w171) -> ("Timestamp"=w170:dbl)
          }
          frame "m1m3_logevent_RejectedForces" {
            n105 = control-ref of="logevent_RejectedForces"() -> (w179:refnum<vi>)
            n106 = local read "logevent_RejectedForces"() -> (w176:T5)
            n107 = call "GetEventRejectedForcesField.vi"("Event Data"=w178, "Cluster in"=w179) -> ("Array"=w177:string[])  [unwired: 9 in]
            n108 = Unbundle By Name(w176) -> ("Timestamp"=w175:dbl)
          }
          frame "m1m3_logevent_RejectedOffsetForces" {
            n109 = control-ref of="logevent_RejectedOffsetForces"() -> (w184:refnum<vi>)
            n110 = local read "logevent_RejectedOffsetForces"() -> (w181:T4)
            n111 = call "GetEventRejectedOffsetForcesField.vi"("Event Data"=w183, "Cluster in"=w184) -> ("Array"=w182:string[])  [unwired: 9 in]
            n112 = Unbundle By Name(w181) -> ("Timestamp"=w180:dbl)
          }
          frame "m1m3_logevent_RejectedStaticForces" {
            n113 = control-ref of="logevent_RejectedStaticForces"() -> (w189:refnum<vi>)
            n114 = local read "logevent_RejectedStaticForces"() -> (w186:T3)
            n115 = call "GetEventRejectedStaticForcesField.vi"("Event Data"=w188, "Cluster in"=w189) -> ("Array"=w187:string[])  [unwired: 9 in]
            n116 = Unbundle By Name(w186) -> ("Timestamp"=w185:dbl)
          }
          frame "m1m3_logevent_RejectedThermalForces" {
            n117 = control-ref of="logevent_RejectedThermalForces"() -> (w194:refnum<vi>)
            n118 = local read "logevent_RejectedThermalForces"() -> (w191:T2)
            n119 = call "GetEventRejectedThermalForcesField.vi"("Event Data"=w192, "Cluster in"=w194) -> ("Array"=w193:string[])  [unwired: 9 in]
            n120 = Unbundle By Name(w191) -> ("Timestamp"=w190:dbl)
          }
          frame "m1m3_logevent_RejectedVelocityForces" {
            n121 = control-ref of="logevent_RejectedVelocityForces"() -> (w199:refnum<vi>)
            n122 = local read "logevent_RejectedVelocityForces"() -> (w196:T1)
            n123 = call "GetEventRejectedVelocityForcesField.vi"("Event Data"=w198, "Cluster in"=w199) -> ("Array"=w197:string[])  [unwired: 9 in]
            n124 = Unbundle By Name(w196) -> ("Timestamp"=w195:dbl)
          }
        }
        n125 = call "Get Timestamp Cushion.vi"("DoubleTimestampRepresentation"=w43) -> ("TimestampCushion"=w42:dbl)  [unwired: 10 in]
        n126 = call "FAValuesXYZC.vi"("Input"=w45) -> ("Output"=→"Display":string[][])  [unwired: 10 in]
        n127 = To Time Stamp(1:w42) -> (0:→"Timestamp":timestamp)
      }
    }
    n128 = local read "stop"() -> (w39:bool)
  }
  n129 = while {
    stop <- w200 stop-if-true
    n130 = event shown="[1] \"Topic\": Value Change" {
      selector: _ -> [_ _]
      dyn-events: _ -> [_ _]
      timeout: 100 -> [_ _]
      event Timeout {
        n131 = event-data() -> ()  [unwired: 1 in, 3 out]
      }
      event "Topic": Value Change {
        n132 = event-data() -> ()  [unwired: 1 in, 6 out]
        n133 = local read "Topic"() -> (w202:string)
        n134 = case shown="\"m1m3_ForceActuatorData\"" w202 {
          tunnel: [string[] [] ("Array") w205 w210 w215 w220 w225 w230 w235 w240 w245 w250 w255 w260 w265 w270 w275 w280 w285 w290 w295 w300 w305 w310 w315 w320 w325 w330 w335 w340 w345 w350] -> w203
          frame "", Default {
          }
          frame "m1m3_ForceActuatorData" {
            n135 = control-ref of="ForceActuatorData"() -> (w207:refnum<vi>)
            n136 = property class="Clust (strict)"(reference=w207) -> ("Controls[]"=w206:refnum<vi>[])  [unwired: 1 in, 2 out]
            n137 = for {
              tunnel: w206 -> [w209] mode=indexing
              tunnel: [w208] -> w205 mode=indexing
              n138 = property class="Ctl"(reference=w209) -> ("Label.Text"=w208:string)  [unwired: 1 in, 2 out]
            }
          }
          frame "m1m3_logevent_ForceActuatorInfo" {
            n139 = control-ref of="logevent_ForceActuatorInfo"() -> (w211:refnum<vi>)
            n140 = property class="Clust (strict)"(reference=w211) -> ("Controls[]"=w212:refnum<vi>[])  [unwired: 1 in, 2 out]
            n141 = for {
              tunnel: w212 -> [w214] mode=indexing
              tunnel: [w213] -> w210 mode=indexing
              n142 = property class="Ctl"(reference=w214) -> ("Label.Text"=w213:string)  [unwired: 1 in, 2 out]
            }
          }
          frame "m1m3_logevent_ForceActuatorState" {
            n143 = control-ref of="logevent_ForceActuatorState"() -> (w216:refnum<vi>)
            n144 = property class="Clust (strict)"(reference=w216) -> ("Controls[]"=w217:refnum<vi>[])  [unwired: 1 in, 2 out]
            n145 = for {
              tunnel: w217 -> [w219] mode=indexing
              tunnel: [w218] -> w215 mode=indexing
              n146 = property class="Ctl"(reference=w219) -> ("Label.Text"=w218:string)  [unwired: 1 in, 2 out]
            }
          }
          frame "m1m3_logevent_ForceActuatorWarning" {
            n147 = control-ref of="logevent_ForceActuatorWarning"() -> (w221:refnum<vi>)
            n148 = property class="Clust (strict)"(reference=w221) -> ("Controls[]"=w222:refnum<vi>[])  [unwired: 1 in, 2 out]
            n149 = for {
              tunnel: w222 -> [w224] mode=indexing
              tunnel: [w223] -> w220 mode=indexing
              n150 = property class="Ctl"(reference=w224) -> ("Label.Text"=w223:string)  [unwired: 1 in, 2 out]
            }
          }
          frame "m1m3_logevent_ForceSetpointWarning" {
            n151 = control-ref of="logevent_ForceSetpointWarning"() -> (w226:refnum<vi>)
            n152 = property class="Clust (strict)"(reference=w226) -> ("Controls[]"=w227:refnum<vi>[])  [unwired: 1 in, 2 out]
            n153 = for {
              tunnel: w227 -> [w229] mode=indexing
              tunnel: [w228] -> w225 mode=indexing
              n154 = property class="Ctl"(reference=w229) -> ("Label.Text"=w228:string)  [unwired: 1 in, 2 out]
            }
          }
          frame "m1m3_logevent_ForceActuatorForceWarning" {
            n155 = control-ref of="logevent_ForceActuatorForceWarning"() -> (w231:refnum<vi>)
            n156 = property class="Clust (strict)"(reference=w231) -> ("Controls[]"=w232:refnum<vi>[])  [unwired: 1 in, 2 out]
            n157 = for {
              tunnel: w232 -> [w234] mode=indexing
              tunnel: [w233] -> w230 mode=indexing
              n158 = property class="Ctl"(reference=w234) -> ("Label.Text"=w233:string)  [unwired: 1 in, 2 out]
            }
          }
          frame "m1m3_logevent_AppliedAberrationForces" {
            n159 = control-ref of="logevent_AppliedAberrationForces"() -> (w236:refnum<vi>)
            n160 = property class="Clust (strict)"(reference=w236) -> ("Controls[]"=w237:refnum<vi>[])  [unwired: 1 in, 2 out]
            n161 = for {
              tunnel: w237 -> [w239] mode=indexing
              tunnel: [w238] -> w235 mode=indexing
              n162 = property class="Ctl"(reference=w239) -> ("Label.Text"=w238:string)  [unwired: 1 in, 2 out]
            }
          }
          frame "m1m3_logevent_AppliedAccelerationForces" {
            n163 = control-ref of="logevent_AppliedAccelerationForces"() -> (w241:refnum<vi>)
            n164 = property class="Clust (strict)"(reference=w241) -> ("Controls[]"=w242:refnum<vi>[])  [unwired: 1 in, 2 out]
            n165 = for {
              tunnel: w242 -> [w244] mode=indexing
              tunnel: [w243] -> w240 mode=indexing
              n166 = property class="Ctl"(reference=w244) -> ("Label.Text"=w243:string)  [unwired: 1 in, 2 out]
            }
          }
          frame "m1m3_logevent_AppliedActiveOpticForces" {
            n167 = control-ref of="logevent_AppliedActiveOpticForces"() -> (w246:refnum<vi>)
            n168 = property class="Clust (strict)"(reference=w246) -> ("Controls[]"=w247:refnum<vi>[])  [unwired: 1 in, 2 out]
            n169 = for {
              tunnel: w247 -> [w249] mode=indexing
              tunnel: [w248] -> w245 mode=indexing
              n170 = property class="Ctl"(reference=w249) -> ("Label.Text"=w248:string)  [unwired: 1 in, 2 out]
            }
          }
          frame "m1m3_logevent_AppliedAzimuthForces" {
            n171 = control-ref of="logevent_AppliedAzimuthForces"() -> (w251:refnum<vi>)
            n172 = property class="Clust (strict)"(reference=w251) -> ("Controls[]"=w252:refnum<vi>[])  [unwired: 1 in, 2 out]
            n173 = for {
              tunnel: w252 -> [w254] mode=indexing
              tunnel: [w253] -> w250 mode=indexing
              n174 = property class="Ctl"(reference=w254) -> ("Label.Text"=w253:string)  [unwired: 1 in, 2 out]
            }
          }
          frame "m1m3_logevent_AppliedBalanceForces" {
            n175 = control-ref of="logevent_AppliedBalanceForces"() -> (w256:refnum<vi>)
            n176 = property class="Clust (strict)"(reference=w256) -> ("Controls[]"=w257:refnum<vi>[])  [unwired: 1 in, 2 out]
            n177 = for {
              tunnel: w257 -> [w259] mode=indexing
              tunnel: [w258] -> w255 mode=indexing
              n178 = property class="Ctl"(reference=w259) -> ("Label.Text"=w258:string)  [unwired: 1 in, 2 out]
            }
          }
          frame "m1m3_logevent_AppliedCylinderForces" {
            n179 = control-ref of="logevent_AppliedCylinderForces"() -> (w261:refnum<vi>)
            n180 = property class="Clust (strict)"(reference=w261) -> ("Controls[]"=w262:refnum<vi>[])  [unwired: 1 in, 2 out]
            n181 = for {
              tunnel: w262 -> [w264] mode=indexing
              tunnel: [w263] -> w260 mode=indexing
              n182 = property class="Ctl"(reference=w264) -> ("Label.Text"=w263:string)  [unwired: 1 in, 2 out]
            }
          }
          frame "m1m3_logevent_AppliedElevationForces" {
            n183 = control-ref of="logevent_AppliedElevationForces"() -> (w266:refnum<vi>)
            n184 = property class="Clust (strict)"(reference=w266) -> ("Controls[]"=w267:refnum<vi>[])  [unwired: 1 in, 2 out]
            n185 = for {
              tunnel: w267 -> [w269] mode=indexing
              tunnel: [w268] -> w265 mode=indexing
              n186 = property class="Ctl"(reference=w269) -> ("Label.Text"=w268:string)  [unwired: 1 in, 2 out]
            }
          }
          frame "m1m3_logevent_AppliedForces" {
            n187 = control-ref of="logevent_AppliedForces"() -> (w271:refnum<vi>)
            n188 = property class="Clust (strict)"(reference=w271) -> ("Controls[]"=w272:refnum<vi>[])  [unwired: 1 in, 2 out]
            n189 = for {
              tunnel: w272 -> [w274] mode=indexing
              tunnel: [w273] -> w270 mode=indexing
              n190 = property class="Ctl"(reference=w274) -> ("Label.Text"=w273:string)  [unwired: 1 in, 2 out]
            }
          }
          frame "m1m3_logevent_AppliedOffsetForces" {
            n191 = control-ref of="logevent_AppliedOffsetForces"() -> (w276:refnum<vi>)
            n192 = property class="Clust (strict)"(reference=w276) -> ("Controls[]"=w277:refnum<vi>[])  [unwired: 1 in, 2 out]
            n193 = for {
              tunnel: w277 -> [w279] mode=indexing
              tunnel: [w278] -> w275 mode=indexing
              n194 = property class="Ctl"(reference=w279) -> ("Label.Text"=w278:string)  [unwired: 1 in, 2 out]
            }
          }
          frame "m1m3_logevent_AppliedStaticForces" {
            n195 = control-ref of="logevent_AppliedStaticForces"() -> (w281:refnum<vi>)
            n196 = property class="Clust (strict)"(reference=w281) -> ("Controls[]"=w282:refnum<vi>[])  [unwired: 1 in, 2 out]
            n197 = for {
              tunnel: w282 -> [w284] mode=indexing
              tunnel: [w283] -> w280 mode=indexing
              n198 = property class="Ctl"(reference=w284) -> ("Label.Text"=w283:string)  [unwired: 1 in, 2 out]
            }
          }
          frame "m1m3_logevent_AppliedThermalForces" {
            n199 = control-ref of="logevent_AppliedThermalForces"() -> (w286:refnum<vi>)
            n200 = property class="Clust (strict)"(reference=w286) -> ("Controls[]"=w287:refnum<vi>[])  [unwired: 1 in, 2 out]
            n201 = for {
              tunnel: w287 -> [w289] mode=indexing
              tunnel: [w288] -> w285 mode=indexing
              n202 = property class="Ctl"(reference=w289) -> ("Label.Text"=w288:string)  [unwired: 1 in, 2 out]
            }
          }
          frame "m1m3_logevent_AppliedVelocityForces" {
            n203 = control-ref of="logevent_AppliedVelocityForces"() -> (w291:refnum<vi>)
            n204 = property class="Clust (strict)"(reference=w291) -> ("Controls[]"=w292:refnum<vi>[])  [unwired: 1 in, 2 out]
            n205 = for {
              tunnel: w292 -> [w294] mode=indexing
              tunnel: [w293] -> w290 mode=indexing
              n206 = property class="Ctl"(reference=w294) -> ("Label.Text"=w293:string)  [unwired: 1 in, 2 out]
            }
          }
          frame "m1m3_logevent_RejectedAberrationForces" {
            n207 = control-ref of="logevent_RejectedAberrationForces"() -> (w296:refnum<vi>)
            n208 = property class="Clust (strict)"(reference=w296) -> ("Controls[]"=w297:refnum<vi>[])  [unwired: 1 in, 2 out]
            n209 = for {
              tunnel: w297 -> [w299] mode=indexing
              tunnel: [w298] -> w295 mode=indexing
              n210 = property class="Ctl"(reference=w299) -> ("Label.Text"=w298:string)  [unwired: 1 in, 2 out]
            }
          }
          frame "m1m3_logevent_RejectedAccelerationForces" {
            n211 = control-ref of="logevent_RejectedAccelerationForces"() -> (w301:refnum<vi>)
            n212 = property class="Clust (strict)"(reference=w301) -> ("Controls[]"=w302:refnum<vi>[])  [unwired: 1 in, 2 out]
            n213 = for {
              tunnel: w302 -> [w304] mode=indexing
              tunnel: [w303] -> w300 mode=indexing
              n214 = property class="Ctl"(reference=w304) -> ("Label.Text"=w303:string)  [unwired: 1 in, 2 out]
            }
          }
          frame "m1m3_logevent_RejectedActiveOpticForces" {
            n215 = control-ref of="logevent_RejectedActiveOpticForces"() -> (w306:refnum<vi>)
            n216 = property class="Clust (strict)"(reference=w306) -> ("Controls[]"=w307:refnum<vi>[])  [unwired: 1 in, 2 out]
            n217 = for {
              tunnel: w307 -> [w309] mode=indexing
              tunnel: [w308] -> w305 mode=indexing
              n218 = property class="Ctl"(reference=w309) -> ("Label.Text"=w308:string)  [unwired: 1 in, 2 out]
            }
          }
          frame "m1m3_logevent_RejectedAzimuthForces" {
            n219 = control-ref of="logevent_RejectedAzimuthForces"() -> (w311:refnum<vi>)
            n220 = property class="Clust (strict)"(reference=w311) -> ("Controls[]"=w312:refnum<vi>[])  [unwired: 1 in, 2 out]
            n221 = for {
              tunnel: w312 -> [w314] mode=indexing
              tunnel: [w313] -> w310 mode=indexing
              n222 = property class="Ctl"(reference=w314) -> ("Label.Text"=w313:string)  [unwired: 1 in, 2 out]
            }
          }
          frame "m1m3_logevent_RejectedBalanceForces" {
            n223 = control-ref of="logevent_RejectedBalanceForces"() -> (w316:refnum<vi>)
            n224 = property class="Clust (strict)"(reference=w316) -> ("Controls[]"=w317:refnum<vi>[])  [unwired: 1 in, 2 out]
            n225 = for {
              tunnel: w317 -> [w319] mode=indexing
              tunnel: [w318] -> w315 mode=indexing
              n226 = property class="Ctl"(reference=w319) -> ("Label.Text"=w318:string)  [unwired: 1 in, 2 out]
            }
          }
          frame "m1m3_logevent_RejectedCylinderForces" {
            n227 = control-ref of="logevent_RejectedCylinderForces"() -> (w321:refnum<vi>)
            n228 = property class="Clust (strict)"(reference=w321) -> ("Controls[]"=w322:refnum<vi>[])  [unwired: 1 in, 2 out]
            n229 = for {
              tunnel: w322 -> [w324] mode=indexing
              tunnel: [w323] -> w320 mode=indexing
              n230 = property class="Ctl"(reference=w324) -> ("Label.Text"=w323:string)  [unwired: 1 in, 2 out]
            }
          }
          frame "m1m3_logevent_RejectedElevationForces" {
            n231 = control-ref of="logevent_RejectedElevationForces"() -> (w326:refnum<vi>)
            n232 = property class="Clust (strict)"(reference=w326) -> ("Controls[]"=w327:refnum<vi>[])  [unwired: 1 in, 2 out]
            n233 = for {
              tunnel: w327 -> [w329] mode=indexing
              tunnel: [w328] -> w325 mode=indexing
              n234 = property class="Ctl"(reference=w329) -> ("Label.Text"=w328:string)  [unwired: 1 in, 2 out]
            }
          }
          frame "m1m3_logevent_RejectedForces" {
            n235 = control-ref of="logevent_RejectedForces"() -> (w331:refnum<vi>)
            n236 = property class="Clust (strict)"(reference=w331) -> ("Controls[]"=w332:refnum<vi>[])  [unwired: 1 in, 2 out]
            n237 = for {
              tunnel: w332 -> [w334] mode=indexing
              tunnel: [w333] -> w330 mode=indexing
              n238 = property class="Ctl"(reference=w334) -> ("Label.Text"=w333:string)  [unwired: 1 in, 2 out]
            }
          }
          frame "m1m3_logevent_RejectedOffsetForces" {
            n239 = control-ref of="logevent_RejectedOffsetForces"() -> (w336:refnum<vi>)
            n240 = property class="Clust (strict)"(reference=w336) -> ("Controls[]"=w337:refnum<vi>[])  [unwired: 1 in, 2 out]
            n241 = for {
              tunnel: w337 -> [w339] mode=indexing
              tunnel: [w338] -> w335 mode=indexing
              n242 = property class="Ctl"(reference=w339) -> ("Label.Text"=w338:string)  [unwired: 1 in, 2 out]
            }
          }
          frame "m1m3_logevent_RejectedStaticForces" {
            n243 = control-ref of="logevent_RejectedStaticForces"() -> (w341:refnum<vi>)
            n244 = property class="Clust (strict)"(reference=w341) -> ("Controls[]"=w342:refnum<vi>[])  [unwired: 1 in, 2 out]
            n245 = for {
              tunnel: w342 -> [w344] mode=indexing
              tunnel: [w343] -> w340 mode=indexing
              n246 = property class="Ctl"(reference=w344) -> ("Label.Text"=w343:string)  [unwired: 1 in, 2 out]
            }
          }
          frame "m1m3_logevent_RejectedThermalForces" {
            n247 = control-ref of="logevent_RejectedThermalForces"() -> (w346:refnum<vi>)
            n248 = property class="Clust (strict)"(reference=w346) -> ("Controls[]"=w347:refnum<vi>[])  [unwired: 1 in, 2 out]
            n249 = for {
              tunnel: w347 -> [w349] mode=indexing
              tunnel: [w348] -> w345 mode=indexing
              n250 = property class="Ctl"(reference=w349) -> ("Label.Text"=w348:string)  [unwired: 1 in, 2 out]
            }
          }
          frame "m1m3_logevent_RejectedVelocityForces" {
            n251 = control-ref of="logevent_RejectedVelocityForces"() -> (w351:refnum<vi>)
            n252 = property class="Clust (strict)"(reference=w351) -> ("Controls[]"=w352:refnum<vi>[])  [unwired: 1 in, 2 out]
            n253 = for {
              tunnel: w352 -> [w354] mode=indexing
              tunnel: [w353] -> w350 mode=indexing
              n254 = property class="Ctl"(reference=w354) -> ("Label.Text"=w353:string)  [unwired: 1 in, 2 out]
            }
          }
        }
        n255 = property on="Field" class="CmbBox"("Strings[]"=w203) -> ()  [unwired: 2 in, 2 out]
      }
    }
    n256 = local read "stop"() -> (w200:bool)
  }
  n257 = call "GetM1M3SupportEvents.vi"("Model in"="Model in") -> ("M1M3 Support Events out"=w36:refnum<class "M1M3 Support Events.lvclass">)  [unwired: 8 in, 2 out]
  n258 = call "Get M1M3 Support Events.vi"("M1M3 Support Events in"=w36) -> ("M1M3 Support Events"=w37:T31)  [unwired: 9 in, 1 out]
  n259 = Unbundle By Name(w37) -> ("Detailed State Event"=w35:refnum<user-event>, "FA Data"=w34:refnum<user-event>, "FA Info Event"=w31:refnum<user-event>, "FA Force Warning Event"=w30:refnum<user-event>, "FA Warning Event"=w28:refnum<user-event>, "FA State Event"=w29:refnum<user-event>, "Applied AberrationForces Event"=w27:refnum<user-event>, "Applied Acceleration Forcces Event"=w26:refnum<user-event>, "Applied Azimuth Forces Event"=w25:refnum<user-event>, "Applied Active Optic Forces Event"=w24:refnum<user-event>, "Applied Balance Forces Event"=w23:refnum<user-event>, "Applied Cylinder Forces Event"=w22:refnum<user-event>, "Applied Elevation Forces Event"=w21:refnum<user-event>, "Applied Forces Event"=w20:refnum<user-event>, "Applied Offset Forces Event"=w19:refnum<user-event>, "Applied Static Forces Event"=w18:refnum<user-event>, "Applied Thermal Forces Event"=w17:refnum<user-event>, "Applied Velocity Forces Event"=w16:refnum<user-event>, "Rejected Aberration Force Event"=w15:refnum<user-event>, "Rejected Acceleration Forces Event"=w14:refnum<user-event>, "Rejected Active Optic Forces Event"=w13:refnum<user-event>, "Rejected Azimuth Forces Event"=w12:refnum<user-event>, "Rejected Balance Forces Event"=w11:refnum<user-event>, "Rejected Cylinder Forces Event"=w10:refnum<user-event>, "Rejected Elevation Forces Event"=w9:refnum<user-event>, "Rejected Forces Event"=w8:refnum<user-event>, "Rejected Offset Forces Event"=w7:refnum<user-event>, "Rejected Static Forces Event"=w6:refnum<user-event>, "Rejected Thermal Forces Event"=w5:refnum<user-event>, "Rejected Velocity Forces Event"=w4:refnum<user-event>, "Force Setpoint Warning Event"=w1:refnum<user-event>)
  n260 = register-events(w35, w34, w31, w30, w28, w29, w27, w26, w25, w24, w23, w22, w21, w20, w19, w18, w17, w16, w15, w14, w13, w12, w11, w10, w9, w8, w7, w6, w5, w4, w1) -> (reference out=w3:refnum<event-registration>)  [unwired: 2 in, 1 out]
  n261 = flat-sequence {
    tunnel: w3 -> [w356]
    tunnel: [w356] -> w2
    frame #0 {
      n262 = local write "stop"(FALSE ("stop")) -> ()
    }
  }
  n263 = while {
    tunnel: w2 -> [w360]
    tunnel: [w359] -> w33
    i -> [w357]
    stop <- w358 stop-if-true
    n264 = event shown="[1] <FA Data>: User Event" {
      selector: w360 -> [_ _ _]
      dyn-events: [_ _ _] -> w359
      timeout: _ -> [_ _ _]
      tunnel: [w363 FALSE _] -> w358
      tunnel: w357 -> [_ w365 _]
      event User Event {
        n265 = event-data() -> ("logevent_DetailedState.DetailedState"=w362:T32)  [unwired: 1 in]
        n266 = Equal?(x=w362, y=T32."DetailedState_DetailedStates_OfflineState") -> (x = y?=w363:bool)
      }
      event User Event {
        n267 = event-data() -> ("ForceActuatorData"=→"ForceActuatorData":T30)  [unwired: 1 in]
        "Numeric" <- w365
      }
      event User Event {
        n268 = event-data() -> ("logevent_ForceActuatorInfo"=→"logevent_ForceActuatorInfo":T29)  [unwired: 1 in]
      }
    }
    "stop" <- w358
  }
  n269 = Unregister For Events(event registration refnum=w33) -> (error out=w32:errorcluster)  [unwired: 1 in]
  n270 = call <vilib>:"Simple Error Handler.vi"("error in (no error)"=w32) -> ()  [unwired: 4 in, 5 out]
